vi "Datos Out.vi"() -> ()   [LabVIEW 2019]
panel:
  out "DATOS DE PIEZA":T1
  out "Salidas Manuales":T2
  in  "Datos Out":T3
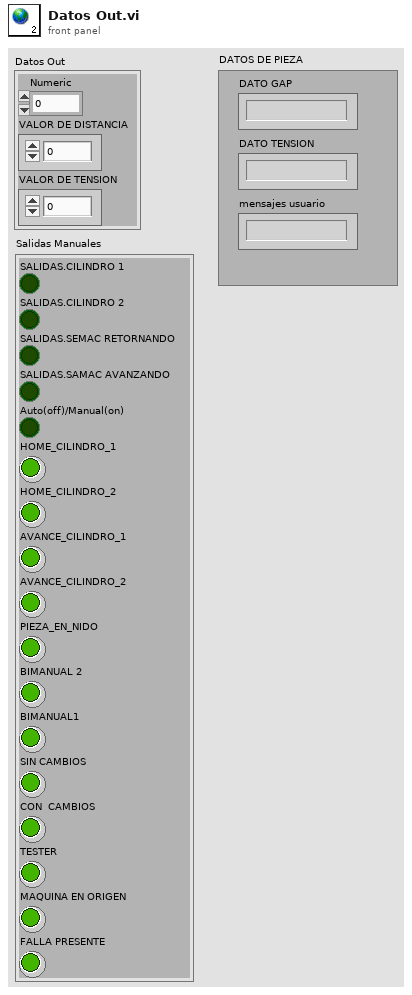
[diagram p1: front panel]
types:
  T1 = cluster{"DATO GAP":string, "DATO TENSION":string, "mensajes usuario":string}
  T2 = cluster{"SALIDAS.CILINDRO 1":bool, "SALIDAS.CILINDRO 2":bool, "SALIDAS.SEMAC RETORNANDO":bool, "SALIDAS.SAMAC AVANZANDO":bool, "Auto(off)/Manual(on)":bool, "HOME_CILINDRO_1":bool, "HOME_CILINDRO_2":bool, "AVANCE_CILINDRO_1":bool, "AVANCE_CILINDRO_2":bool, "PIEZA_EN_NIDO":bool, "BIMANUAL 2":bool, "BIMANUAL1":bool, "SIN CAMBIOS":bool, "CON  CAMBIOS":bool, "TESTER":bool, "MAQUINA EN ORIGEN":bool, "FALLA PRESENTE":bool}
  T3 = cluster{"Numeric":dbl, "VALOR DE DISTANCIA":dbl, "VALOR DE TENSION":dbl}
diagram:
